vi "Piegraphs in Analytics.vi"(5 "values":dbl[](array[numeric])=[14.47, 14.47, 14.68, 14.29, 14.38, 13.88, 13.8], 6 "Colors":u32[](array[numeric]), 7 "Defect Names":string[](array[string]), 8 "error in (no error)":errorcluster, 9 "Defect Values":dbl[](array[numeric])=[14.47, 14.47, 14.68, 14.29, 14.38, 13.88, 13.8], 10 "Draw Area Size":T1={"Width"=500, "Height"=200}, 11 "Defect Statistics":refnum<vi>) -> (0 "error out":errorcluster, 2 "Names with %  values":string[](array[string]), 3 "Labels":picture)   [LabVIEW 2019, in "Zen Analytics.lvlib" / "Zen Analytics.lvclass"]
uses:
  Zen Analytics.lvclass
  <vilib>/Utility/miscctls.llb/LVBoundsTypeDef.ctl
panel:
  out "Value":i32
types:
  T1 = typedef "LVBoundsTypeDef.ctl" = cluster{"Width":u32, "Height":u32}
  T2 = cluster{"left":i16, "top":i16, "right":i16, "bottom":i16}
  T3 = cluster{"Font Name:":string, "Size":i16, "Strikeout?":bool, "Italic?":bool, "Underline?":bool, "Outline?":bool, "Shadow?":bool, "Bold?":bool}
  T4 = enum16{"None", "Stacked", "Clockwise", "Counterclockwise"}
  T5 = enum16{"User-specified Font", "Application Font", "System Font", "Dialog Font"}
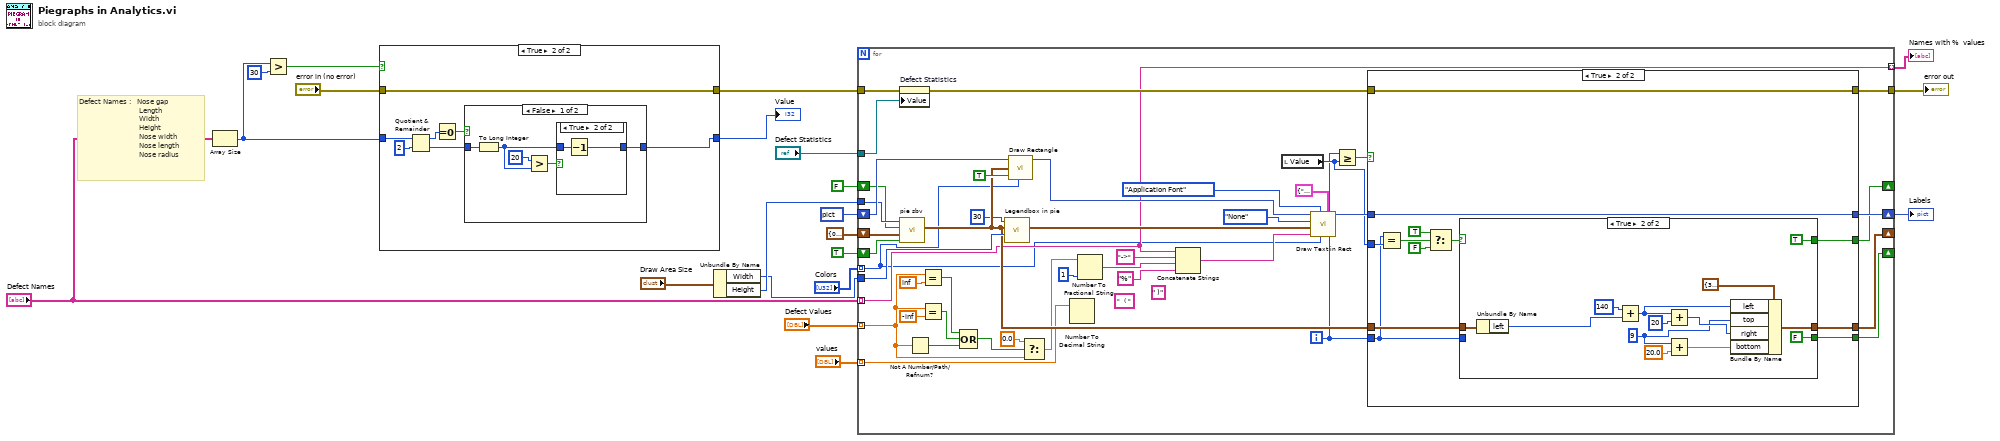
[diagram p0: block diagram]
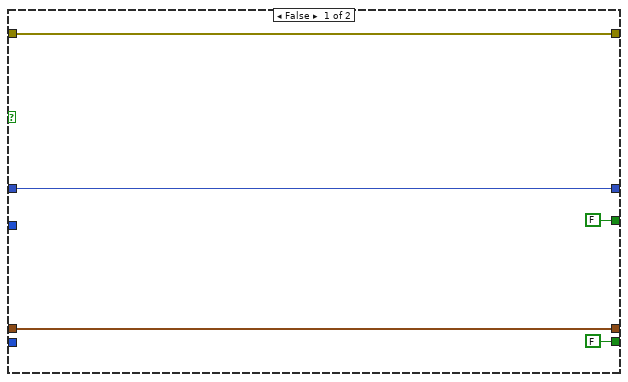
[diagram p2: hidden frame]
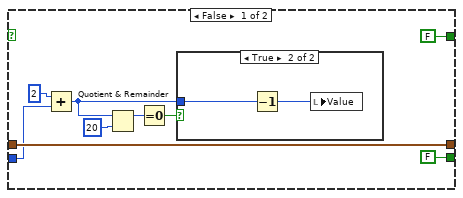
[diagram p3: hidden frame]
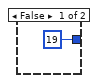
[diagram p6: hidden frame]
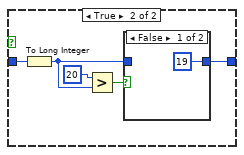
[diagram p7: hidden frame]
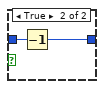
[diagram p8: hidden frame]
diagram:
  # "Defect Names :   Nose gap\n                              Length\n                              Width\n                              Height\n                              Nose width\n                              Nose length\n                              Nose radius"
  n1 = Array Size(array="Defect Names") -> (size(s)=w16:i32)
  n2 = Greater?(x=w16, y=30) -> (0:w18:bool)
  n3 = case shown="True" w18 {
    tunnel: w16 -> [w23 w30]
    tunnel: [w23 w24] -> w17
    tunnel: "error in (no error)" -> [w22 w25]
    tunnel: [w22 w25] -> w21
    frame False {
    }
    frame True {
      n4 = Quotient & Remainder(x=w30, y=2) -> (x-y*floor(x/y)=w26:i32, floor(x/y)=w27:i32)
      n5 = Equal To 0?(x=w26) -> (x = 0?=w28:bool)
      n6 = case shown="False" w28 {
        tunnel: w27 -> [w32 w43]
        tunnel: [w31 w39] -> w24
        frame False {
          n7 = To Long Integer(number=w32) -> (32bit integer=w33:i32)
          n8 = Greater?(x=20 ("y"), y=w33) -> (0:w35:bool)
          n9 = case shown="True" w35 {
            tunnel: [19 w37] -> w31
            tunnel: w33 -> [_ w38]
            frame False {
            }
            frame True {
              n10 = Decrement(x=w38) -> (x-1=w37:i32)
            }
          }
        }
        frame True {
          n11 = To Long Integer(number=w43) -> (32bit integer=w40:i32)
          n12 = Greater?(x=20 ("y"), y=w40) -> (0:w42:bool)
          n13 = case shown="False" w42 {
            tunnel: [19 ("y") w45] -> w39
            tunnel: w40 -> [_ w46]
            frame False {
            }
            frame True {
              n14 = Decrement(x=w46) -> (x-1=w45:i32)
            }
          }
        }
      }
    }
  }
  "Value" <- w17
  n15 = Unbundle By Name("Draw Area Size") -> ("Width"=w11:u32, "Height"=w12:u32)
  n16 = for {
    tunnel: "Defect Names" -> [w53] mode=indexing
    shift-right: [w86] -> w13
    shift-left: picture data[5B] ("new picture") -> [w88]
    shift-right: [w85] -> _
    shift-left: T2 {"left"=0, "top"=0, "right"=0, "bottom"=0} ("rect") -> [w84]
    tunnel: w12 -> [w79]
    tunnel: w11 -> [w77]
    tunnel: "Colors" -> [w47] mode=indexing
    shift-right: [w83] -> _
    shift-left: TRUE ("s") -> [w82]
    shift-right: [w78] -> _
    shift-left: FALSE ("s") -> [w58]
    tunnel: "Defect Values" -> [w63] mode=indexing
    tunnel: [w53] -> w19 mode=indexing
    tunnel: w21 -> [w56]
    tunnel: [w62] -> w1
    tunnel: "Defect Statistics" -> [w54]
    tunnel: "values" -> [w49] mode=indexing
    i -> [w57]
    (unwired) " )" ("string")
    (unwired) "  ( " ("string")
    n17 = property on="Defect Statistics" class="LVObjRef (strict)"(error in=w56, "Value"=w54) -> (error out=w55:errorcluster)  [unwired: 1 in, 1 out]
    n18 = call "pie sbv.vi"("s"=w82, "rect 2"=w84, "Next 1?"=w58, "Height"=w79) -> ("rect"=w76:T2)  [unwired: 7 in]
    n19 = Not A Number/Path/Refnum?(number/path/refnum=w63) -> (NaN/Path/Refnum?=w70:bool)
    n20 = Equal?(x=w63, y=inf) -> (x = y?=w72:bool)
    n21 = Equal?(x=w63, y=-inf) -> (x = y?=w71:bool)
    n22 = Compound Arithmetic op=OR(w72, w71, w70) -> (w69:bool)
    n23 = call "Legendbox in pie.vi"("Width"=w77, "Last Text"=w76, "Gap"=30) -> ("New Text"=w60:T2)  [unwired: 8 in]
    n24 = call <vilib>:"Draw Rectangle.vi"("picture"=w88, "rect"=w76, "fill?(F)"=TRUE, "color(black)"=w47) -> ("new picture"=w89:picture)  [unwired: 5 in]
    n25 = Select(t=0.0, s=w69, f=w63) -> (s? t:f=w67:dbl)
    n26 = Number To Decimal String(number=w49) -> ()  [unwired: 1 in, 1 out]
    n27 = Number To Fractional String(number=w67, precision (6)=i16 1) -> (F-format string=w66:string)  [unwired: 2 in]
    n28 = Concatenate Strings(w53, "->", w66, "%" ("string")) -> (w64:string)
    n29 = local read "Value"() -> (w61:i32)
    n30 = call <vilib>:"Draw Text in Rect.vi"("[user-specified font]"=T3 {"Font Name:"="", "Size"=20, "Strikeout?"=FALSE, "Italic?"=FALSE, "Underline?"=FALSE, "Outline?"=FALSE, "Shadow?"=FALSE, "Bold?"=TRUE}, "text color(black)"=w47, "desired font(Application)"=T5."Application Font", "text"=w64, "rect"=w60, "text orientation"=T4."None", "picture"=w89) -> ("new picture"=w87:picture)  [unwired: 1 in, 3 out]
    n31 = Greater Or Equal?(x=w57, y=w61) -> (x >= y?=w80:bool)
    n32 = case shown="True" w80 {
      tunnel: w87 -> [w94 w106]
      tunnel: [w94 w106] -> w86
      tunnel: w76 -> [w93 w102]
      tunnel: [w93 w103] -> w85
      tunnel: [FALSE ("s") w100] -> w83
      tunnel: w57 -> [_ w96]
      tunnel: [FALSE ("s") w99] -> w78
      tunnel: w61 -> [_ w98]
      tunnel: [w90 w95] -> w62
      tunnel: w55 -> [w90 w95]
      frame False {
      }
      frame True {
        n33 = Equal?(x=w96, y=w98) -> (x = y?=w101:bool)
        n34 = Select(t=TRUE ("s"), s=w101, f=FALSE) -> (s? t:f=w97:bool)
        n35 = case shown="True" w97 {
          tunnel: [w115 w129] -> w103
          tunnel: w102 -> [w115 w124]
          tunnel: [FALSE ("s") FALSE ("s")] -> w100
          tunnel: [FALSE ("s") TRUE ("s")] -> w99
          tunnel: w96 -> [w109 _]
          frame False {
            n36 = Add(x=2, y=w109) -> (x+y=w108:i32)
            n37 = Quotient & Remainder(x=w108, y=20) -> (x-y*floor(x/y)=w111:i32)  [unwired: 1 out]
            n38 = Equal To 0?(x=w111) -> (x = 0?=w110:bool)
            n39 = case shown="True" w110 {
              tunnel: w108 -> [_ w117]
              frame False {
              }
              frame True {
                n40 = Decrement(x=w117) -> (x-1=w116:i32)
                n41 = local write "Value"(w116) -> ()
              }
            }
          }
          frame True {
            w118 = i16 9 ("x")
            n42 = Unbundle By Name(w124) -> ("left"=w123:i16)
            n43 = Add(x=i16 140, y=w123) -> (x+y=w121:i16)
            n44 = Add(x=w121, y=i16 20) -> (x+y=w119:i16)
            n45 = Add(x=w118, y=20.0) -> (x+y=w127:dbl)
            n46 = Bundle By Name(cluster=T2 {"left"=30, "top"=0, "right"=30, "bottom"=0} ("rect 2"), "left"=w121, "top"=w118, "right"=w119, "bottom"=w127) -> (w129:T2)
          }
        }
      }
    }
  }
  "error out" <- w1
  "Names with %  values" <- w19
  "Labels" <- w13
